vi "IMAQ FPGA CXP Pixel Buffer 8-Bit x 8.vi"(7 "Reset":bool, 8 "Read":bool, 9 "Tap":u8=8, 10 "Valid Bytes":u8, 11 "Pixel Data In U8x32":u8[](array[numeric])=[0, 0, 0, 0, 0, 0, 0, 0, 0, 0, 0, 0, 0, 0, 0, 0, 0, 0, 0, 0, 0, 0, 0, 0, 0, 0, 0, 0, 0, 0, 0, 0]) -> (2 "#Elements Read":u8, 3 "Pixel Data Out U8x8":u8[](array[numeric]))   [LabVIEW 2020]
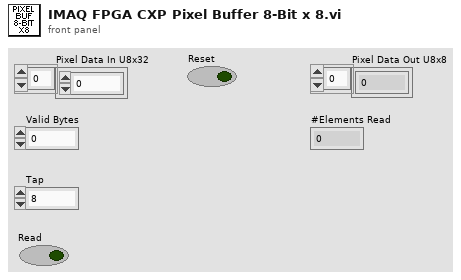
[diagram p1: front panel]
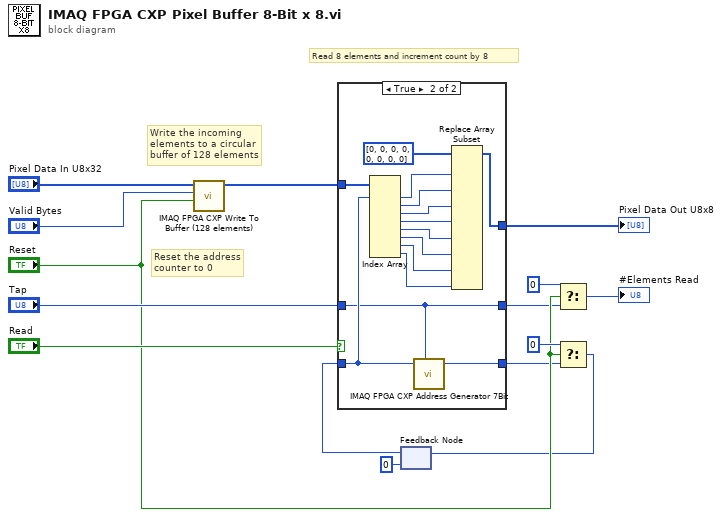
[diagram p0: block diagram]
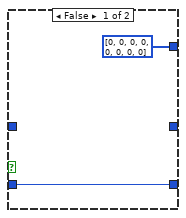
[diagram p2: hidden frame]
diagram:
  # "Reset the address\ncounter to 0"
  # "Write the incoming\nelements to a circular\nbuffer of 128 elements"
  # "Read 8 elements and increment count by 8"
  n1 = call <vilib>:"IMAQ FPGA CXP Write To Buffer (128 elements).vi"("Reset"="Reset", "Valid Bytes"="Valid Bytes", "Pixel Data In U8x32"="Pixel Data In U8x32") -> ("Buffer Out"=w14:u8[])  [unwired: 8 in]
  n2 = feedback #1(u8 0 ("y")) -> (w13:u8)
  n3 = case shown="True" "Read" {
    tunnel: w14 -> [_ w31]
    tunnel: [_ w19] -> w4
    tunnel: [u8[] [0, 0, 0, 0, 0, 0, 0, 0] w29] -> w12
    tunnel: [w17 w18] -> w3
    tunnel: w13 -> [w17 w20]
    tunnel: "Tap" -> [_ w19]
    frame False {
    }
    frame True {
      n4 = Index Array(array=w31, index #1=w20) -> (element #1=w28:u8, element #2=w27:u8, element #3=w26:u8, element #4=w25:u8, element #5=w24:u8, element #6=w23:u8, element #7=w22:u8, element #8=w21:u8)  [unwired: 7 in]
      n5 = call <vilib>:"IMAQ FPGA CXP Address Generator 7Bit.vi"("Base Address"=w20, "Index"=w19) -> ("Address Out"=w18:u8)  [unwired: 7 in]
      n6 = Replace Array Subset(array=u8[] [0, 0, 0, 0, 0, 0, 0, 0], new element #1=w28, new element #2=w27, new element #3=w26, new element #4=w25, new element #5=w24, new element #6=w23, new element #7=w22, new element #8=w21) -> (w29:u8[])  [unwired: 8 in]
    }
  }
  "Pixel Data Out U8x8" <- w12
  n7 = Select(t=u8 0 ("Tap"), s="Reset", f=w4) -> (s? t:f=→"#Elements Read":u8)
  n8 = Select(t=u8 0 ("y"), s="Reset", f=w3) -> (s? t:f=w2:u8)
  n9 = feedback-in #1(w2) -> ()
